vi "get Fcurve segments.vi"(0 "reference in":refnum<class "Fcurve.lvclass">, 5 "error in (no error)":errorcluster) -> (14 "reference out":refnum<class "Fcurve.lvclass">, 18 "Fcurve Segment data":cluster{"X":dbl[], "Y":dbl[]}[](array[cluster]), 19 "error out":errorcluster)   [LabVIEW 2019, in "Fcurve.lvclass"]
uses:
  Fcurve.lvclass
  Fcurve sections.ctl
  Segment MaxMin --cluster.ctl
  <vilib>/Waveform/WDTOps.llb/WDT Get Waveform Subset DBL.vi
panel:
  out "Actual seg duration":cluster{"Start":i32, "Duration":i32}[](array[cluster])
  out "Segment duration (S)":dbl[](array[numeric]) format="%0.2f"
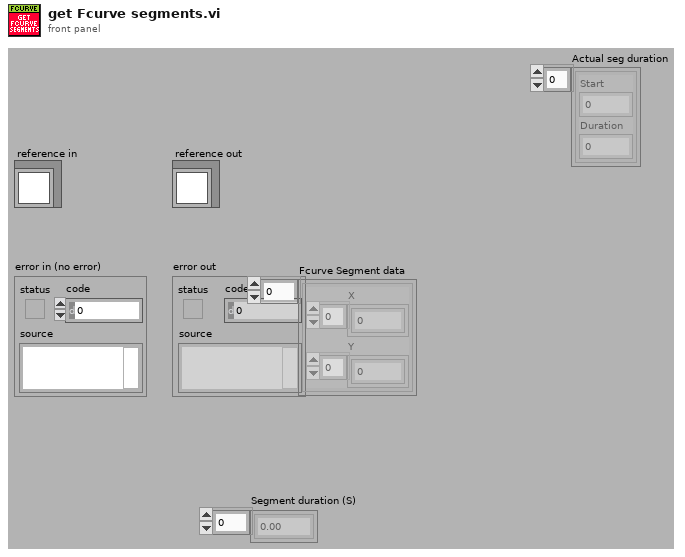
[diagram p1: front panel]
types:
  T1 = typedef "Fcurve.lvclass/Fcurve sections.ctl" = enum16{"Approach", "Contact", "Retract"}
  T2 = typedef "Fcurve.lvclass/Segment MaxMin --cluster.ctl" = cluster{"Def":cluster{"max value":dbl, "min value":dbl}, "Zpos":cluster{"max value":dbl, "min value":dbl}}
  T3 = typedef "Fcurve.lvclass/ObjectAttributesRef.ctl" = refnum<data-value>
  T4 = typedef "Fcurve.lvclass/ObjectAttributes.ctl" = cluster{"MyAttribute":dbl, "Fcurve Metadata":T5, "Contact Spread of dev":dbl, "Tau Delay (ms)":dbl, "Points of contact":dbl, "Def_wfm":cluster{"Max":dbl, "Min":dbl}, "Zpos_wfm":cluster{"Max":dbl, "Min":dbl}, "Contact stat?":bool, "Real AI dt (s)":dbl, "Decimation":cluster{"App":cluster{"Dec":i32, "apply":bool}, "Con":cluster{"Dec":i32, "apply":bool}, "Ret":cluster{"Dec":i32, "apply":bool}}, "Segment def[0]":dbl, "Segment Zpos[0]":dbl, "Raw Datum":waveform(dbl)[], "Group metadata":T6, "M_data obj":refnum<class "metadata.lvclass">, "Channel name(s)":string[], "Segment fcurve data":cluster{"X":dbl[], "Y":dbl[]}[], "Segment duration":cluster{"Start":i32, "Duration":i32}[], "Segment info":T7[], "Segment durations (S)":dbl[], "Segments Maxmin":T2[]}
  T5 = typedef "Fcurve.lvclass/Metadata.ctl" = cluster{"dt (us)":dbl, "Dec Factor":dbl, "Z piezo Sensitivity (nm/V)":dbl, "K (N/m)":dbl, "Sp (V)":dbl, "Contact (ms)":dbl, "Zpos contact":dbl, "Vel_app (nm/s)":dbl, "Vel_ret (nm/s)":dbl, "deltaV (nm)":dbl, "Def_V0 (v)":dbl, "Piezo gain":dbl, "invOLS (nm/V)":dbl}
  T6 = typedef "TDMS_DataHandler.lvclass/Fcurve Meta data.ctl" = cluster{"property names":string[], "property values":variant[]}
  T7 = typedef "Fcurve.lvclass/Fcurve segments --cluster.ctl" = cluster{"type":T8, "nb points":i32, "dec factor":u32, "sampling rate (S/s)":u32}
  T8 = typedef "metadata.lvclass/Segment type--combobox.ctl" = string
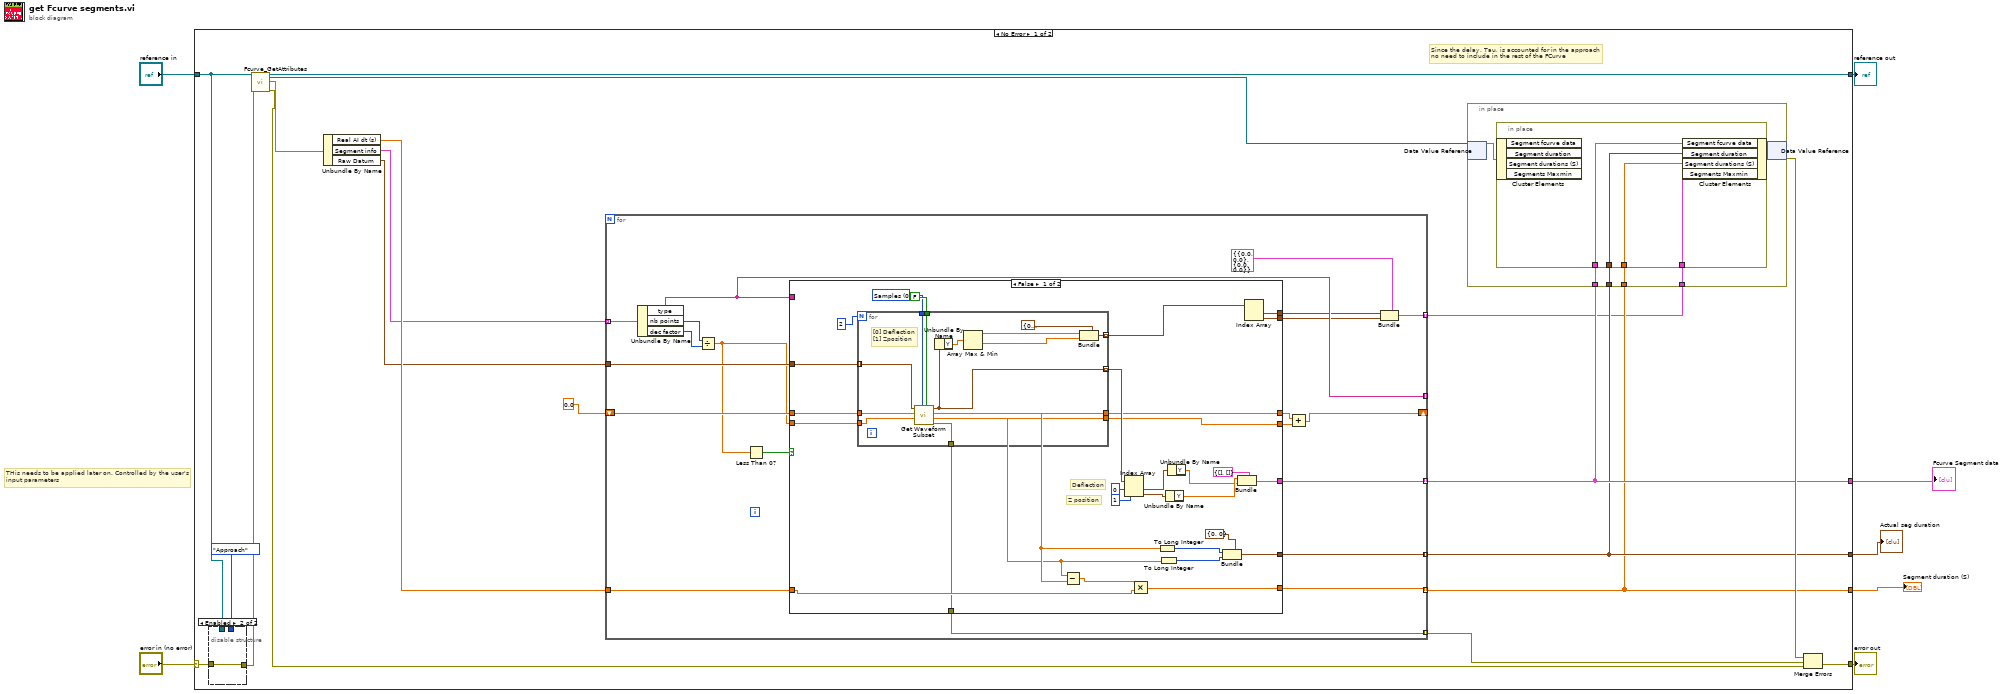
[diagram p0: block diagram]
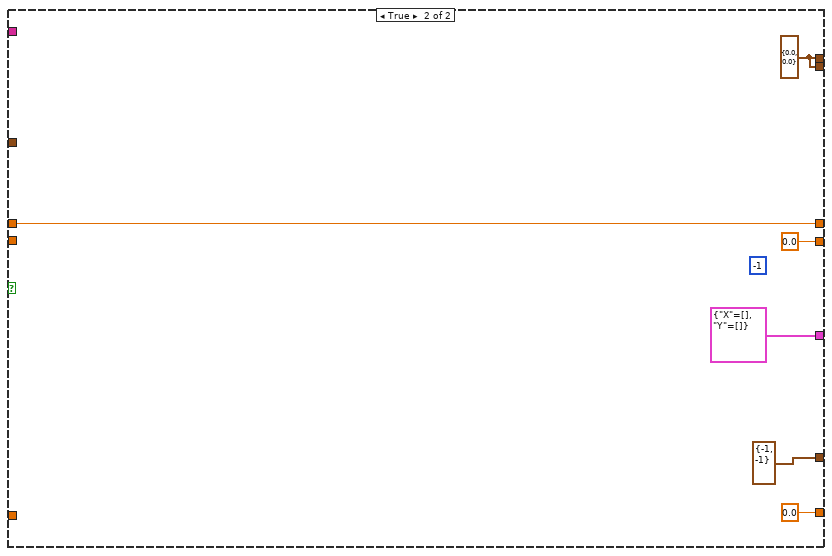
[diagram p2: hidden frame]
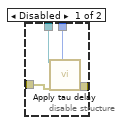
[diagram p3: hidden frame]
diagram:
  # "THis needs to be applied later on. Controlled by the user's\ninput parameters"
  n1 = case shown="No Error" "error in (no error)" {
    selector: "error in (no error)" -> [w22 w111]
    tunnel: [w26 w111] -> w6
    tunnel: [w25 w110] -> w4
    tunnel: "reference in" -> [w23 w110]
    tunnel: [w13 _] -> w2
    tunnel: [w14 _] -> w3
    tunnel: [w10 _] -> w1
    frame No Error {
      # "Since the delay, Tau, is accounted for in the approach\nno need to include in the rest of the FCurve"
      n2 = disable-structure shown="Enabled" {
        disable-tunnel: w23 -> [w98 _]
        disable-tunnel: w22 -> [w97 w99]
        disable-tunnel: [w96 w99] -> w21
        disable-tunnel: Fcurve_sections."Approach" ("Section") -> [w95 _]
        frame Disabled {
          n3 = call "Apply tau delay.vi"("reference in"=w98, "error in (no error)"=w97, "Section"=w95) -> ("error out"=w96:errorcluster)  [unwired: 13 in, 3 out]
        }
        frame Enabled {
        }
      }
      n4 = call "Fcurve_GetAttributes.vi"("reference in"=w23, "error in (no error)"=w21) -> ("reference out"=w25:refnum<class "Fcurve.lvclass">, "attributes ref"=w15:T3, "attributes"=w24:T4, "error out"=w20:errorcluster)  [unwired: 14 in]
      n5 = Unbundle By Name(w24) -> ("Real AI dt (s)"=w18:dbl, "Segment info"=w12:T7[], "Raw Datum"=w8:waveform(dbl)[])
      n6 = for {
        tunnel: [w35] -> w19 mode=indexing
        tunnel: [w44] -> w14 mode=indexing
        tunnel: [w43] -> w13 mode=indexing
        tunnel: w12 -> [w42] mode=indexing
        tunnel: [w34] -> _ mode=indexing
        shift-right: [w27] -> _
        shift-left: 0.0 ("start samples/time") -> [w40]
        tunnel: w8 -> [w41]
        tunnel: w18 -> [w45]
        tunnel: [w46] -> w10 mode=indexing
        tunnel: [w31] -> w9 mode=indexing
        n7 = Unbundle By Name(w42) -> ("type"=w34:T8, "nb points"=w39:i32, "dec factor"=w38:u32)
        n8 = Divide(x=w39, y=w38) -> (x/y=w37:dbl)
        n9 = Less Than 0?(x=w37) -> (x < 0?=w36:bool)
        n10 = case shown="False" w36 {
          tunnel: [w74 0.0] -> w46
          tunnel: [w51 _] -> w35
          tunnel: w45 -> [w62 _]
          tunnel: [w60 cluster{"X":dbl[], "Y":dbl[]} {"X"=[], "Y"=[]} ("Fcurve.Approach")] -> w44
          tunnel: [w59 cluster{"Start":i32, "Duration":i32} {"Start"=-1, "Duration"=-1} ("Fcurve index.Contact indices")] -> w43
          tunnel: w41 -> [w58 _]
          tunnel: w40 -> [w57 w94]
          tunnel: [w54 w94] -> w29
          tunnel: w37 -> [w52 _]
          tunnel: w34 -> [_ _]
          tunnel: [w49 w90] -> w33
          tunnel: [w48 w90] -> w32
          tunnel: [w47 0.0 ("actual duration")] -> w28
          frame False {
            w55 = u16 0 items=["Samples", "Relative Time"] ("start/duration format")
            # "Z position"
            # "Deflection"
            n11 = for {
              N: 2 -> [_]
              tunnel: [w88] -> w47
              tunnel: [w80] -> w72 mode=indexing
              tunnel: w58 -> [w87] mode=indexing
              tunnel: [w86] -> w54
              tunnel: [w85] -> w51
              tunnel: w57 -> [w84]
              tunnel: FALSE ("open interval? (T)") -> [w83]
              tunnel: w55 -> [w82]
              tunnel: w52 -> [w81]
              tunnel: [w75] -> w50 mode=indexing
              # "[0] Deflection\n[1] Zposition"
              n12 = call-poly <vilib>:"Get Waveform Subset.vi"("open interval? (T)"=w83, "start/duration format"=w82, "duration"=w81, "start samples/time"=w84, "waveform in"=w87) -> ("error out"=w85:errorcluster, "actual duration"=w88:dbl, "actual start samples/time"=w86:dbl, "waveform out"=w80:waveform(dbl))  [unwired: 1 in]
              n13 = Unbundle By Name(w80) -> ("Y"=w79:dbl[])
              n14 = Array Max & Min(array=w79) -> (max value=w78:dbl, min value=w77:dbl)  [unwired: 2 out]
              n15 = Bundle(cluster=cluster{"max value":dbl, "min value":dbl} {"max value"=0.0, "min value"=0.0} ("Def"), "max value"=w78, "min value"=w77) -> (w75:cluster{"max value":dbl, "min value":dbl})
            }
            n16 = Subtract(x=w47, y=w54) -> (x-y=w53:dbl)
            n17 = Index Array(array=w72, index #1=0 ("index"), index #2=1 ("index")) -> (element #1=w71:waveform(dbl), element #2=w70:waveform(dbl))
            n18 = Multiply(x=w53, y=w62) -> (x*y=w74:dbl)
            n19 = To Long Integer(number=w54) -> (32bit integer=w68:i32)
            n20 = To Long Integer(number=w47) -> (32bit integer=w69:i32)
            n21 = Unbundle By Name(w70) -> ("Y"=w65:dbl[])
            n22 = Unbundle By Name(w71) -> ("Y"=w64:dbl[])
            n23 = Bundle(cluster=cluster{"Start":i32, "Duration":i32} {"Start"=0, "Duration"=0} ("Fcurve index.Contact indices"), "Start"=w68, "Duration"=w69) -> (w59:cluster{"Start":i32, "Duration":i32})
            n24 = Bundle(cluster=cluster{"X":dbl[], "Y":dbl[]} {"X"=[], "Y"=[]} ("Fcurve.Approach"), "X"=w65, "Y"=w64) -> (w60:cluster{"X":dbl[], "Y":dbl[]})
            n25 = Index Array(array=w50) -> (element #1=w49:cluster{"max value":dbl, "min value":dbl}, element #2=w48:cluster{"max value":dbl, "min value":dbl})  [unwired: 2 in]
          }
          frame True {
            w90 = cluster{"max value":dbl, "min value":dbl} {"max value"=0.0, "min value"=0.0} ("Def")
            (unwired) -1
          }
        }
        n26 = Add(x=w29, y=w28) -> (x+y=w27:dbl)
        n27 = Bundle(cluster=T2 {"Def"={"max value"=0.0, "min value"=0.0}, "Zpos"={"max value"=0.0, "min value"=0.0}} ("Segment MaxMin"), "Def"=w33, "Zpos"=w32) -> (w31:T2)
      }
      n28 = in-place {
        in-place-border: w14 -> [w103]
        in-place-border: w13 -> [w102]
        in-place-border: w10 -> [w101]
        in-place-border: w9 -> [w100]
        n29 = in-place-dvr #1(w15) -> (w104:T4)  [unwired: 1 out]
        n30 = in-place {
          in-place-border: w103 -> [w109]
          in-place-border: w102 -> [w108]
          in-place-border: w101 -> [w107]
          in-place-border: w100 -> [w106]
          n31 = in-place-cluster #2(w104) -> ()  [unwired: 4 out]
          n32 = in-place-cluster #2("Segment fcurve data"=w109, "Segment duration"=w108, "Segment durations (S)"=w107, "Segments Maxmin"=w106) -> (w105:T4)
        }
        n33 = in-place-dvr #1(w105) -> (w16:errorcluster)  [unwired: 1 out]
      }
      n34 = Merge Errors(w16, w19, w20) -> (w26:errorcluster)
    }
    frame Error {
    }
  }
  "error out" <- w6
  "reference out" <- w4
  "Fcurve Segment data" <- w3
  "Actual seg duration" <- w2
  "Segment duration (S)" <- w1
